vi "215.Get travel range(SubVI).vi"(8 "error in (no error)":errorcluster, 11 "VISA resource name":refnum<visa-resource-name>="COM7") -> (0 "error out":errorcluster, 1 "String":string, 2 "Connected":bool, 3 "VISA Out":refnum<visa-resource-name>)   [LabVIEW 2020]
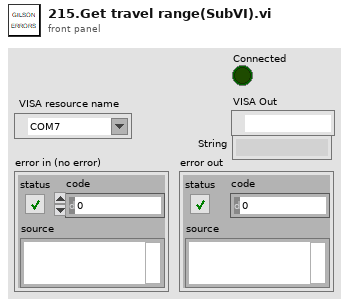
[diagram p1: front panel]
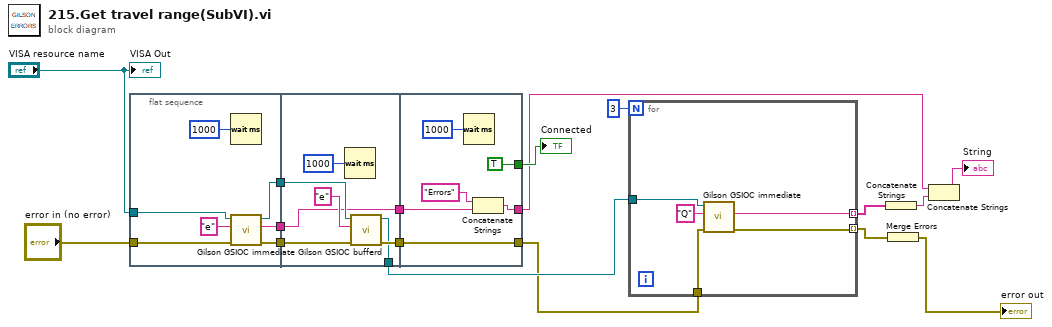
[diagram p0: block diagram]
diagram:
  n1 = flat-sequence {
    tunnel: "VISA resource name" -> [w22]
    tunnel: "error in (no error)" -> [w24]
    tunnel: [w21] -> w17
    tunnel: [w20] -> w16
    tunnel: [w18] -> w14
    tunnel: w17 -> [w31]
    tunnel: w16 -> [w29]
    tunnel: w14 -> [w27]
    tunnel: [w27] -> w11
    tunnel: [w26] -> w10
    tunnel: [w25] -> w8
    tunnel: [TRUE ("Connected")] -> w15
    tunnel: w11 -> [w36]
    tunnel: [w32] -> w7
    tunnel: [w34] -> w2
    tunnel: w10 -> [w32]
    frame #0 {
      n2 = Wait (ms)(milliseconds to wait=u32 1000) -> ()  [unwired: 1 out]
      n3 = call <instrlib>:"Gilson GSIOC immediate.vi"("error in (no error)"=w24, "Immediate command"="e", "VISA resource name"=w22) -> ("error out"=w20:errorcluster, "Receive string"=w18:string, "VISA resource name"=w21:refnum<visa-resource-name>)  [unwired: 6 in]
    }
    frame #1 {
      n4 = Wait (ms)(milliseconds to wait=u32 1000) -> ()  [unwired: 1 out]
      n5 = call <instrlib>:"Gilson GSIOC bufferd.vi"("error in (no error)"=w29, "Bufferd command"="e", "VISA resource name"=w31) -> ("error out"=w26:errorcluster, "VISA resource name out"=w25:refnum<visa-resource-name>)  [unwired: 6 in, 1 out]
    }
    frame #2 {
      n6 = Wait (ms)(milliseconds to wait=u32 1000) -> ()  [unwired: 1 out]
      n7 = Concatenate Strings("Errors" ("string"), w36) -> (w34:string)
    }
  }
  n8 = for {
    N: 3 -> [_]
    tunnel: w8 -> [w41]
    tunnel: w7 -> [w40]
    tunnel: [w39] -> w6 mode=indexing
    tunnel: [w38] -> w4 mode=indexing
    n9 = call <instrlib>:"Gilson GSIOC immediate.vi"("error in (no error)"=w40, "Immediate command"="Q", "VISA resource name"=w41) -> ("error out"=w39:errorcluster, "Receive string"=w38:string)  [unwired: 6 in, 1 out]
  }
  n10 = Concatenate Strings(w4) -> (w3:string)
  n11 = Merge Errors(w6) -> (→"error out":errorcluster)
  n12 = Concatenate Strings(w2, w3) -> (→"String":string)
  "VISA Out" <- "VISA resource name"
  "Connected" <- w15
